vi "Magnetometer - Standalone Main.vi"(8 "error in (no error)":errorcluster) -> ()   [LabVIEW 2021]
uses:
  Lab 5/Lab 5 Code/Heading_TDef.ctl
  <vilib>/Platform/TimedLoop/XDataNode/timing_clust.ctl
  <vilib>/Platform/TimedLoop/XDataNode/nitl_modes.ctl
  <vilib>/Platform/TimedLoop/XDataNode/wakeup.ctl
  <vilib>/myRIO/Instrument Drivers/Onboard IO/I2C/typedefs/I2C User Configuration.ctl
  <vilib>/myRIO/Instrument Drivers/Onboard IO/I2C/typedefs/I2C Transfer Rate.ctl
  <vilib>/Utility/error.llb/Error Cluster From Error Code.vi
  <vilib>/myRIO/Common/Instrument Driver Framework/myRIO v1.0/I2C/vis/myRIO v1.0 Configure I2C.vi
  <vilib>/platform/TimedLoop/XDataNode/XDataNode.xnode
  <vilib>/Platform/TimedLoop/XDataNode/XDNodeRunTimeDep.lvlib
  <vilib>/myRIO/Instrument Drivers/Onboard IO/I2C/I2C.lvlib
panel:
  out "Heading Output (Str)":T1
  out "Magnetometer Flux (uT)":dbl[](array[numeric])
  out "Heading":dbl
  in  "stop":bool
  out "error out":errorcluster
  out "Who am I":u8[](array[numeric])
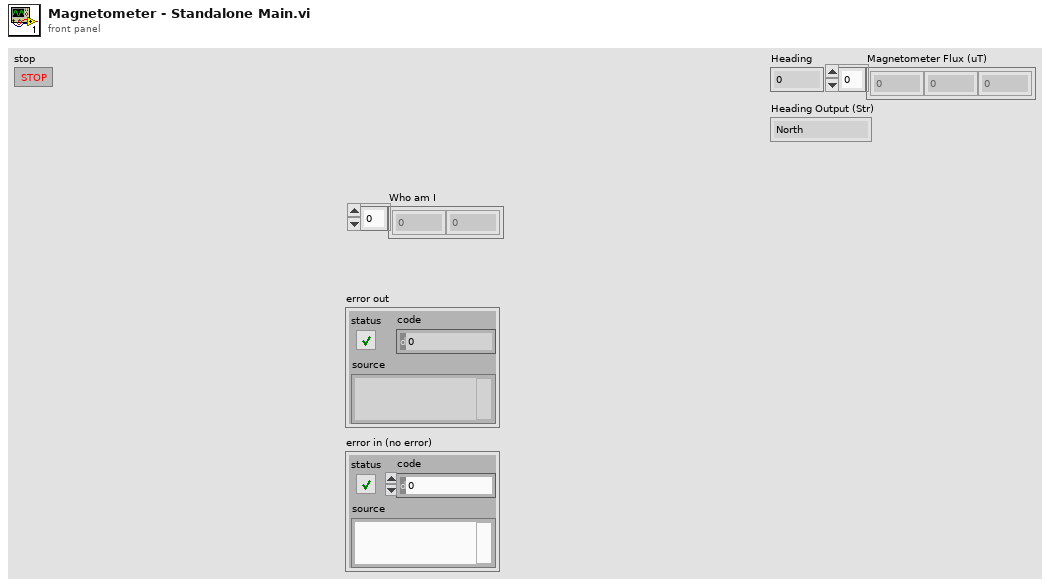
[diagram p1: front panel]
types:
  T1 = typedef "Heading_TDef.ctl" = enum16{"North ", "North East", "East", "Southeast", "South", "Southwest", "West", "Northwest"}
  T2 = typedef "I2C.lvlib/I2C User Configuration.ctl" = cluster{"I2C Transfer Rate":T3}
  T3 = typedef "I2C.lvlib/I2C Transfer Rate.ctl" = enum16{"Standard mode (100 kbps)", "Fast mode (400 kbps)"}
  T4 = typedef "I2C.lvlib/I2C Reference.ctl" = cluster{"myRIO Reference":T5, "I2C Channels Enum":T9, "I2C Configuration":T10}
  T5 = typedef "myRIO Generic Hardware Reference.ctl" = cluster{"myRIO Model":T6, "myRIO Hardware Reference":T7}
  T6 = typedef "Hardware Version Enum.ctl" = enum16{"Unknown", "myRIO-1900", "myRIO-1950", "roboRIO", "NI ELVIS RIO CM", "ELVIS III"}
  T7 = typedef "myRIO v1.0 Reference.ctl" = cluster{"Generic FPGA Reference":T8, "Allow multiple opens":bool}
  T8 = typedef "Generic FPGA Reference.ctl" = refnum<k20>
  T9 = typedef "I2C Channels Enum.ctl" = enum16{"Not Connected", "A/I2C", "B/I2C", "I2C/I2C"}
  T10 = typedef "I2C.lvlib/I2C Configuration.ctl" = cluster{"I2C Transfer Rate":T3}
  T11 = typedef "XDNodeRunTimeDep.lvlib/timing_clust.ctl" = cluster{"Expected End [f-1]":u64, "Actual End [f-1]":u64, "Finished Late? [f-1]":bool, "Expected End [i-1]":u64, "Actual End [i-1]":u64, "Finished Late? [i-1]":bool, "Expected Start [i]":u64, "Actual Start [i]":u64, "Expected Start [f]":u64, "Actual Start [f]":u64, "Source Name":string, "Structure Name":string, "Period":i64, "Deadline":i64, "Offset":i64, "Start":i64, "Priority":i32, "Timeout":i32, "Mode":T12, "Wakeup Reason":T13, "Error":errorcluster, "Source Type":string, "Secondary Source Type":string, "Global End Time":u64, "Global Start Time":u64, "Frame Duration":u64, "Iteration Duration":u64, "Assigned CPU":i32, "I/O Scan Engine Mode":u32}
  T12 = typedef "XDNodeRunTimeDep.lvlib/nitl_modes.ctl" = enum32{"No Change", "Process missed periods, maintain original phase", "Discard missed periods, maintain original phase", "Process missed periods, ignore original phase", "Discard missed periods, ignore original phase"}
  T13 = typedef "XDNodeRunTimeDep.lvlib/wakeup.ctl" = enum32{"Normal", "Aborted", "Asynchronous wakeup", "Timing source error", "Timed loop error", "Timeout"}
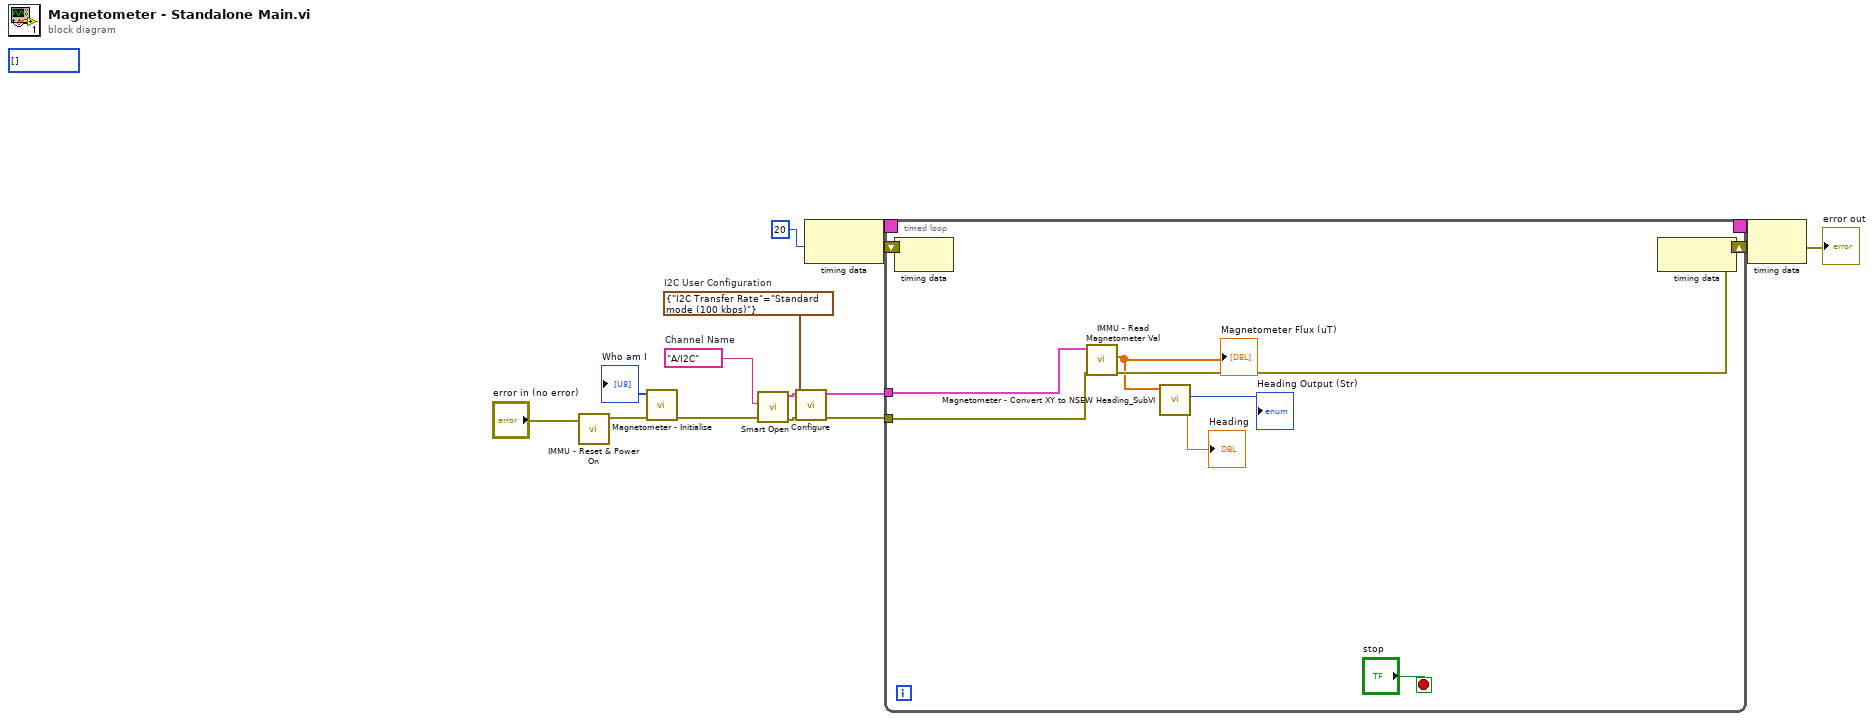
[diagram p0: block diagram]
diagram:
  w6 = T2 {"I2C Transfer Rate"=enum."Standard mode (100 kbps)"}  # I2C User Configuration
  w7 = tag "A/I2C"  # Channel Name
  (unwired) u8[] []
  n1 = call "IMMU - Reset & Power On.vi"("error in (no error)"="error in (no error)") -> ("error out"=w9:errorcluster)  [unwired: 10 in]
  n2 = call "Magnetometer - Initialise.vi"("error in (no error)"=w9) -> ("error out"=w2:errorcluster, "Who am I"=→"Who am I":u8[])  [unwired: 9 in]
  n3 = call <vilib>:"Smart Open.vi"("error in (no error)"=w2, "Channel Name"=w7) -> ("error out"=w4:errorcluster, "I2C Ref Out"=w5:T4)  [unwired: 8 in]
  n4 = call <vilib>:"Configure.vi"("error in (no error)"=w4, "I2C User Configuration"=w6, "I2C Ref In"=w5) -> ("error out"=w1:errorcluster, "I2C Ref Out"=w3:T4)  [unwired: 7 in]
  n5 = node-c288(i64 20 ("Period")) -> (w13:T11)
  n6 = timed-loop {
    timing: w13 -> [_]
    timing-out: [_] -> w12
    shift-right: [w21] -> w14
    shift-left: _ -> [_]
    tunnel: w3 -> [w17]
    tunnel: w1 -> [w16]
    stop <- "stop" stop-if-true
    n7 = node-c288() -> ()  [unwired: 1 in, 1 out]
    n8 = call "IMMU - Read Magnetometer Val.vi"("error in (no error)"=w16, "I2C Ref In"=w17) -> ("error out"=w21:errorcluster, "Magnetometer Flux Out (uT)"=w15:dbl[])  [unwired: 7 in, 1 out]
    "Magnetometer Flux (uT)" <- w15
    n9 = call "Magnetometer - Convert XY to NSEW Heading_SubVI.vi"("Flux In (uT)"=w15) -> ("Heading Output (Str)"=→"Heading Output (Str)":T1, "Heading"=→"Heading":dbl)  [unwired: 9 in]
    n10 = node-c288() -> ()  [unwired: 1 in, 1 out]
  }
  "error out" <- w14
  n11 = node-c288(w12) -> ()  [unwired: 1 out]
